vi "uA_Measurement_kit_v2_logging.vi"() -> ()   [LabVIEW 2015]
uses:
  <vilib>/Utility/file.llb/Write Delimited Spreadsheet (string).vi
panel:
  out "uA":dbl format="%#_4g"
  out "Vbat":dbl format="%#_4g"
  out "current time":timestamp
  in  "Record uA & Vbat":bool
  in  "Path":path
  out "uA 2":dbl(graph)
  out "Vbat Monitor":dbl(graph)
  in  "uA_bank0":dbl=1.5 format="%#_13g"
  out "Task out":refnum<k21>="Stop"
  out "Sample rate":dbl=20000.0 format="%#_13g"
  out "Clear":bool=TRUE
  out "Ver":string
  # "uPower kit V2.1"
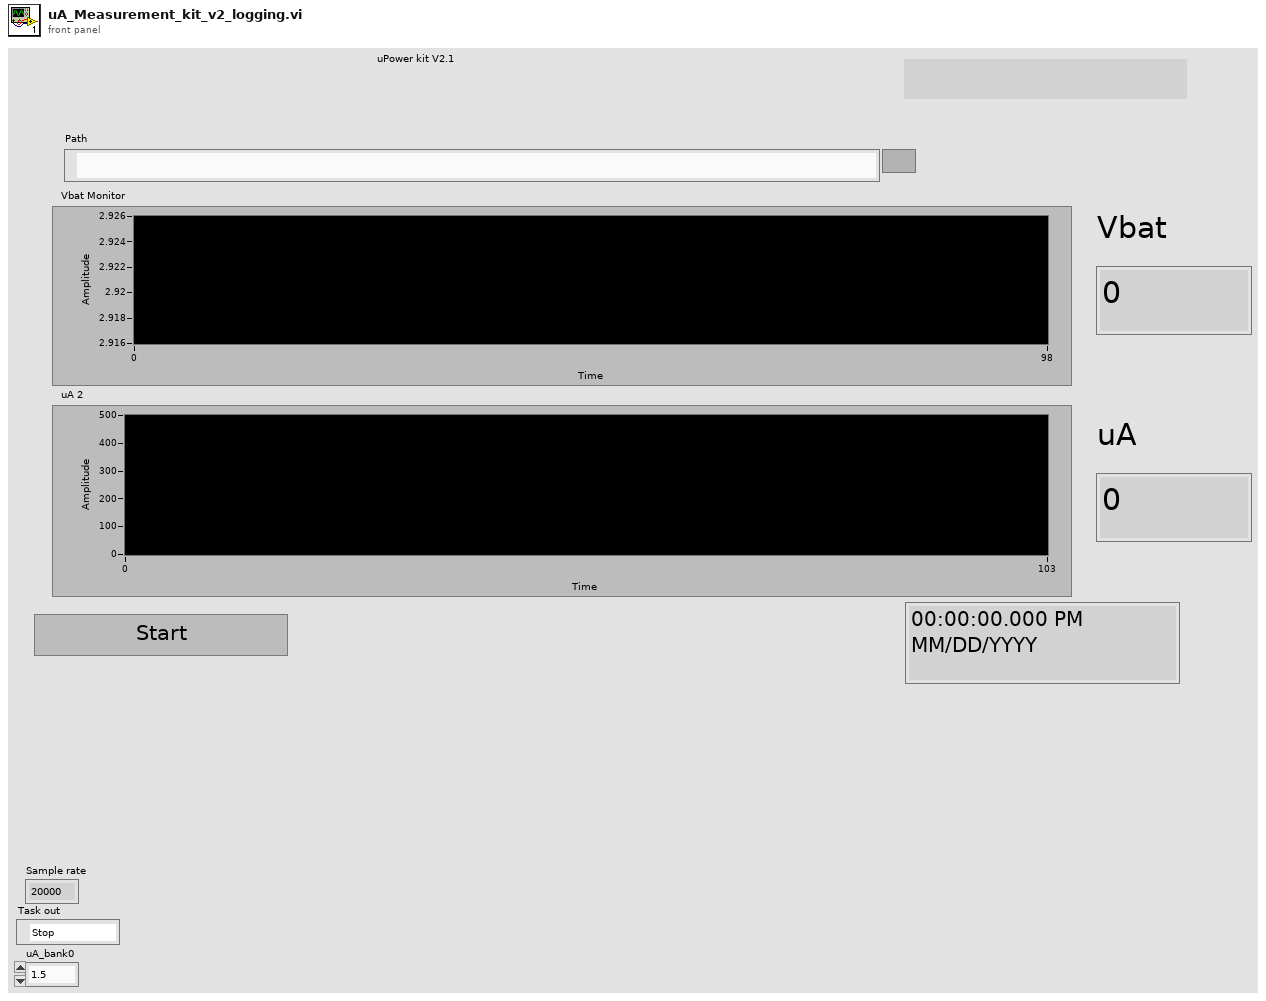
[diagram p1: front panel]
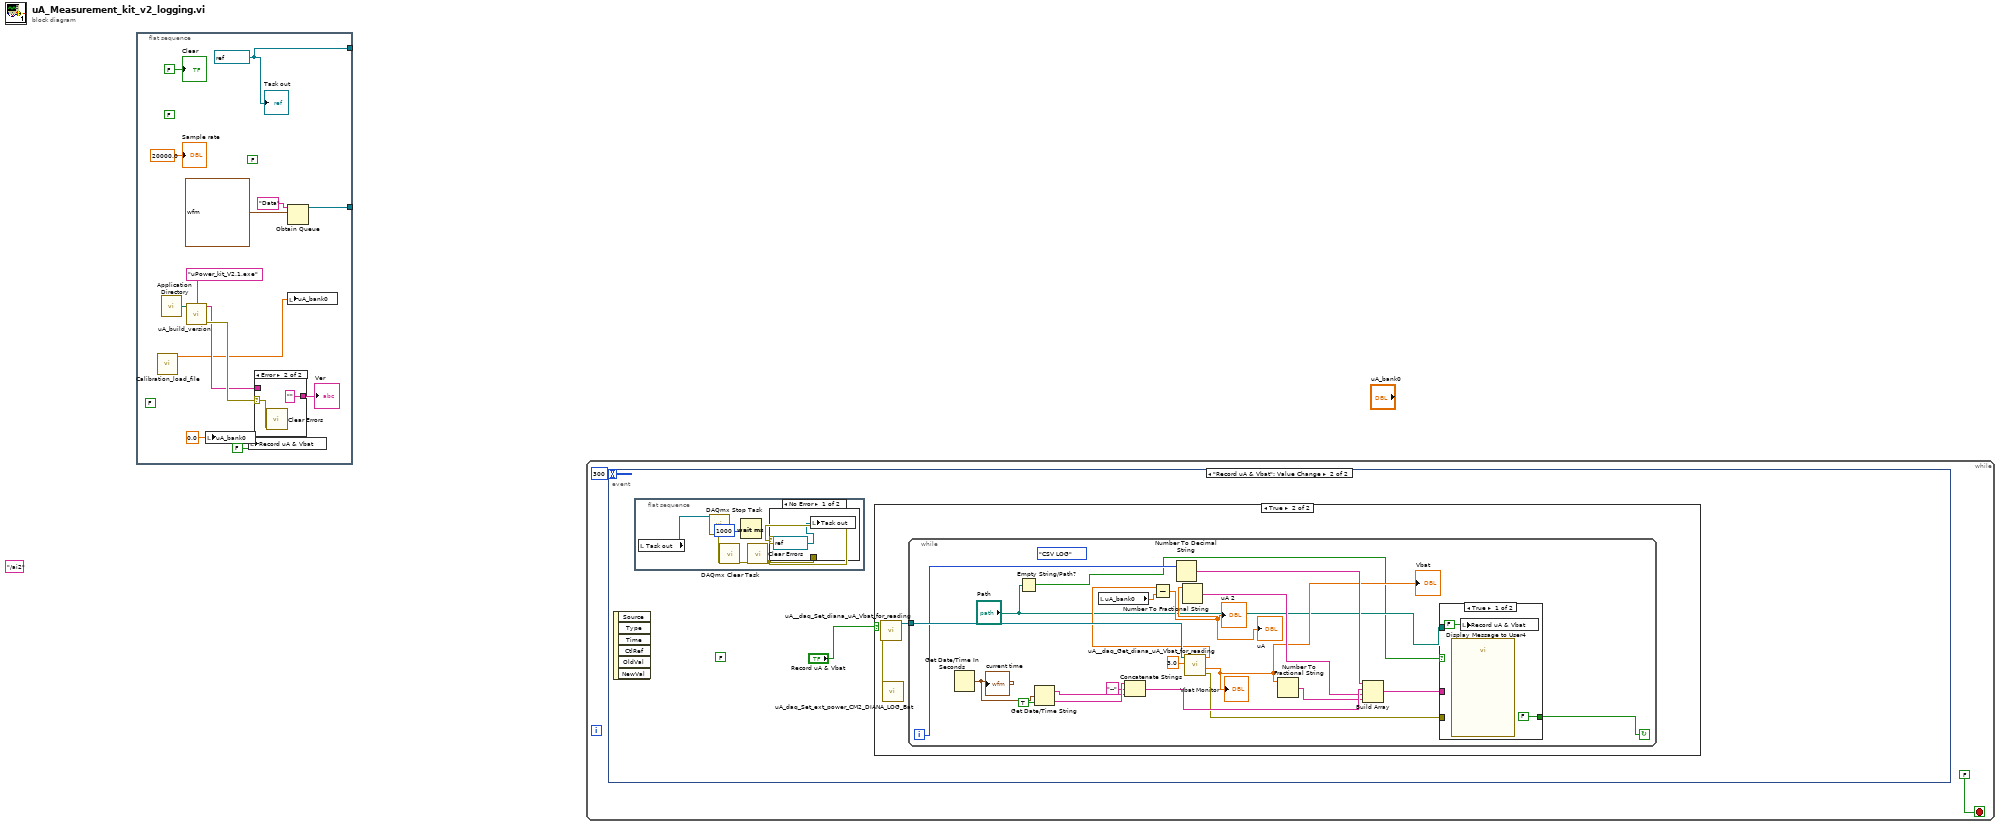
[diagram p0: block diagram]
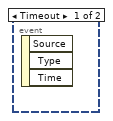
[diagram p3: hidden frame]
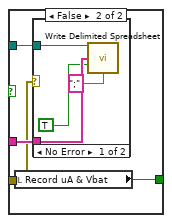
[diagram p6: hidden frame]
diagram:
  (unwired) "/ai2" ("string")
  n1 = flat-sequence {
    tunnel: [w8] -> _
    tunnel: [w10] -> _
    frame #0 {
      (unwired) FALSE ("Power ON/OFF")
      (unwired) FALSE ("Measure")
      (unwired) FALSE ("Visible")
      w8 = refnum<k21> "Stop" ("task out")
      n2 = call "Calibration_load_file.vi"() -> ("uABank0"=w2:dbl)  [unwired: 9 in, 2 out]
      n3 = call <vilib>:"Application Directory.vi"() -> ("Application Directory"=w9:path)
      n4 = call "uA_build_version.vi"("name or relative path"="uPower_kit_V2.1.exe", "path"=w9) -> ("error out"=w7:errorcluster, "FileVersion"=w6:string)  [unwired: 7 in, 1 out]
      n5 = local write "uA_bank0"(0.0 ("uA_calib_0")) -> ()
      n6 = local write "Record uA & Vbat"(FALSE ("Record uA & Vbat")) -> ()
      n7 = case shown="Error" w7 {
        selector: w7 -> [_ w17]
        tunnel: w6 -> [w15 _]
        tunnel: [w15 "" ("FileVersion")] -> w5
        frame No Error {
        }
        frame Error {
          n8 = call <vilib>:"Clear Errors.vi"("error in (no error)"=w17) -> ()  [unwired: 5 in, 2 out]
        }
      }
      "Ver" <- w5
      n9 = Obtain Queue(name (unnamed)="Data", element data type=waveform(sgl) {"t0"=timestamp(0 s since 1904-01-01), "dt"=1.0, "Y"=[]} ("Waveform Chart 2")) -> (queue out=w10:refnum<queue>)  [unwired: 3 in, 2 out]
      n10 = local write "uA_bank0"(w2) -> ()
      "Clear" <- FALSE ("Clear")
      "Sample rate" <- 20000.0 ("Sample rate")
      "Task out" <- w8
    }
  }
  n11 = while {
    stop <- FALSE stop-if-true
    n12 = event shown="[1] \"Record uA & Vbat\": Value Change" {
      selector: _ -> [_ _]
      dyn-events: _ -> [_ _]
      timeout: 300 -> [_ _]
      event Timeout {
        n13 = event-data() -> ()  [unwired: 1 in, 3 out]
      }
      event "Record uA & Vbat": Value Change {
        (unwired) FALSE ("Measure")
        n14 = event-data() -> ()  [unwired: 1 in, 6 out]
        n15 = flat-sequence {
          frame #0 {
            n16 = local read "Task out"() -> (w23:refnum<k21>)
            n17 = call <vilib>:"DAQmx Stop Task.vi"("task/channels in"=w23) -> ("task out"=w22:refnum<k21>, "error out"=w25:errorcluster)  [unwired: 13 in]
            n18 = call <vilib>:"DAQmx Clear Task.vi"("task in"=w22, "error in"=w25) -> ("error out"=w24:errorcluster)  [unwired: 13 in]
            n19 = Wait (ms)(milliseconds to wait=u32 1000) -> ()  [unwired: 1 out]
            n20 = call <vilib>:"Clear Errors.vi"("error in (no error)"=w24) -> ("error out"=w21:errorcluster)  [unwired: 5 in, 1 out]
            n21 = case shown="No Error" w21 {
              tunnel: w21 -> [_ _]
              frame No Error {
                n22 = local write "Task out"(refnum<k21> "Stop" ("y")) -> ()
              }
              frame Error {
              }
            }
          }
        }
        n23 = case shown="True" "Record uA & Vbat" {
          frame False {
          }
          frame True {
            n24 = call "uA_daq_Set_ext_power_CM2_DIANA_LOG_Bat.vi"() -> ("error out"=w30:errorcluster, "USB DAQ out"=w29:tag)  [unwired: 10 in]
            n25 = call "uA__daq_Set_diana_uA_Vbat_for_reading.vi"("error in (no error)"=w30, "USB DAQ in"=w29) -> ("Refnum out"=w28:refnum<k21>)  [unwired: 8 in, 1 out]
            n26 = while {
              tunnel: w28 -> [w51]
              i -> [w41]
              stop <- w31 continue-if-true
              (unwired) enum32{"Current Tracking", "Image", "CSV LOG"}."CSV LOG" ("Tab Control")
              n27 = Get Date/Time In Seconds() -> (seconds since 1Jan1904=w50:timestamp)
              "current time" <- w50
              n28 = Empty String/Path?(string/path="Path") -> (empty?=w32:bool)
              n29 = Get Date/Time String(seconds (now)=w50, want seconds? (F)=TRUE) -> (date string=w48:string, time string=w49:string)  [unwired: 1 in]
              n30 = local read "uA_bank0"() -> (w36:dbl)
              n31 = Concatenate Strings(w49, "--" ("string"), w48) -> (w46:string)
              n32 = Number To Decimal String(number=w41) -> (decimal integer string=w40:string)  [unwired: 1 in]
              n33 = call "uA__daq_Get_diana_uA_Vbat_for_reading.vi"("Coef"=3.0, "Refnum in"=w51) -> ("error out"=w37:errorcluster, "Vbat"=w39:dbl, "uA Current"=w35:dbl)  [unwired: 5 in, 2 out]
              "Vbat Monitor" <- w39
              "Vbat" <- w39
              n34 = Subtract(x=w35, y=w36) -> (x-y=w34:dbl)
              "uA 2" <- w34
              "uA" <- w34
              n35 = Number To Fractional String(number=w34) -> (F-format string=w45:string)  [unwired: 3 in]
              n36 = Number To Fractional String(number=w39) -> (F-format string=w44:string)  [unwired: 3 in]
              n37 = Build Array(w40, w46, w45, w44) -> (w43:string[])
              n38 = case shown="True" w32 {
                tunnel: w43 -> [_ w57]
                tunnel: w37 -> [_ w56]
                tunnel: "Path" -> [_ w55]
                tunnel: [FALSE ("Record uA & Vbat") w54] -> w31
                frame True {
                  n39 = call "Display Message to User4"() -> ()  [unwired: 10 in, 2 out]
                  n40 = local write "Record uA & Vbat"(FALSE ("Record uA & Vbat")) -> ()
                }
                frame False {
                  n41 = local read "Record uA & Vbat"() -> (w54:bool)
                  n42 = case shown="No Error" w56 {
                    tunnel: w57 -> [w61 _]
                    tunnel: w55 -> [w58 _]
                    frame No Error {
                      n43 = call-poly <vilib>:"Write Delimited Spreadsheet.vi"("file path (dialog if empty)"=w58, "1D data"=w61, "append to file? (F)"=TRUE, "delimiter (\\t)"=";" ("delimiter (\\t)")) -> ()  [unwired: 10 in, 2 out]
                    }
                    frame Error {
                    }
                  }
                }
              }
            }
          }
        }
      }
    }
  }
